vi "XYScan - PLC Controler.vi"() -> ()   [LabVIEW 2018]
uses:
  <vilib>/NI/Modbus Library/API/Wrapper/Create Serial Master.vi
  <vilib>/NI/Modbus Library/API/Master/Modbus Master.lvclass
  <vilib>/NI/Modbus Library/API/Wrapper/API Main.lvlib
panel:
  in  "Distance Mode":bool
  out "Step Y Number":i16=50
  in  "Y Auto Distance":i16=100
  in  "X Auto Distance":i16=200
  in  "Y Distance":u32=200
  in  "X Distance":u32=4
  in  "Y Step":dbl=1.0
  in  "Z Distance":i16=10
  in  "Speed":i32=6
  in  "Home":bool
  in  "Z Up":bool
  in  "Z Down":bool
  in  "Y For":bool
  in  "X Left":bool
  in  "Y Back":bool
  in  "X Right":bool
  in  "VISA":refnum<visa-resource-name>="COM12"
  in  "Stop":bool
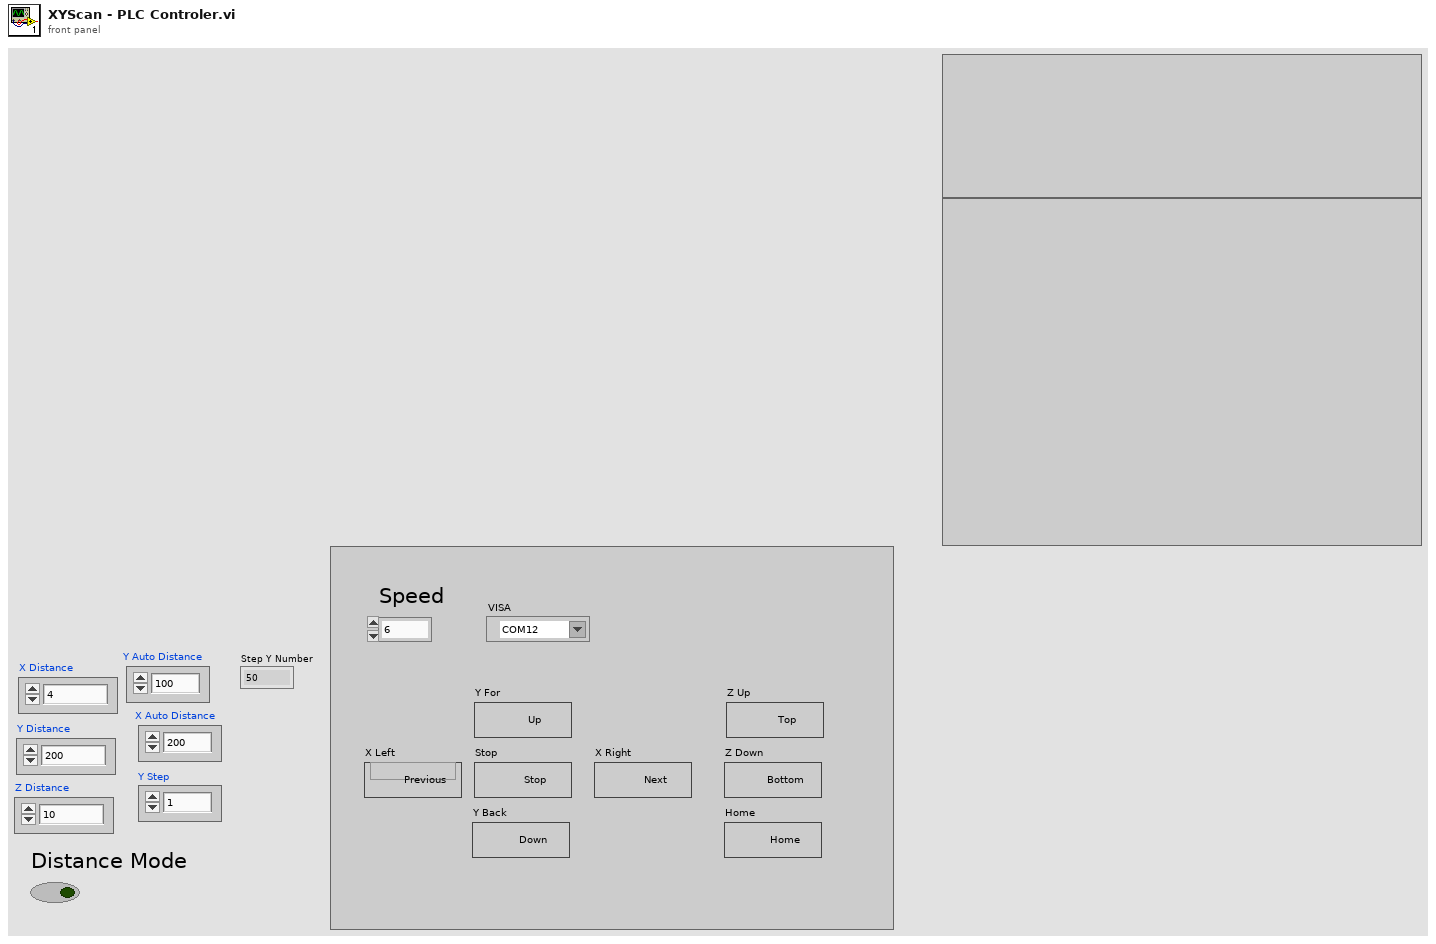
[diagram p1: front panel]
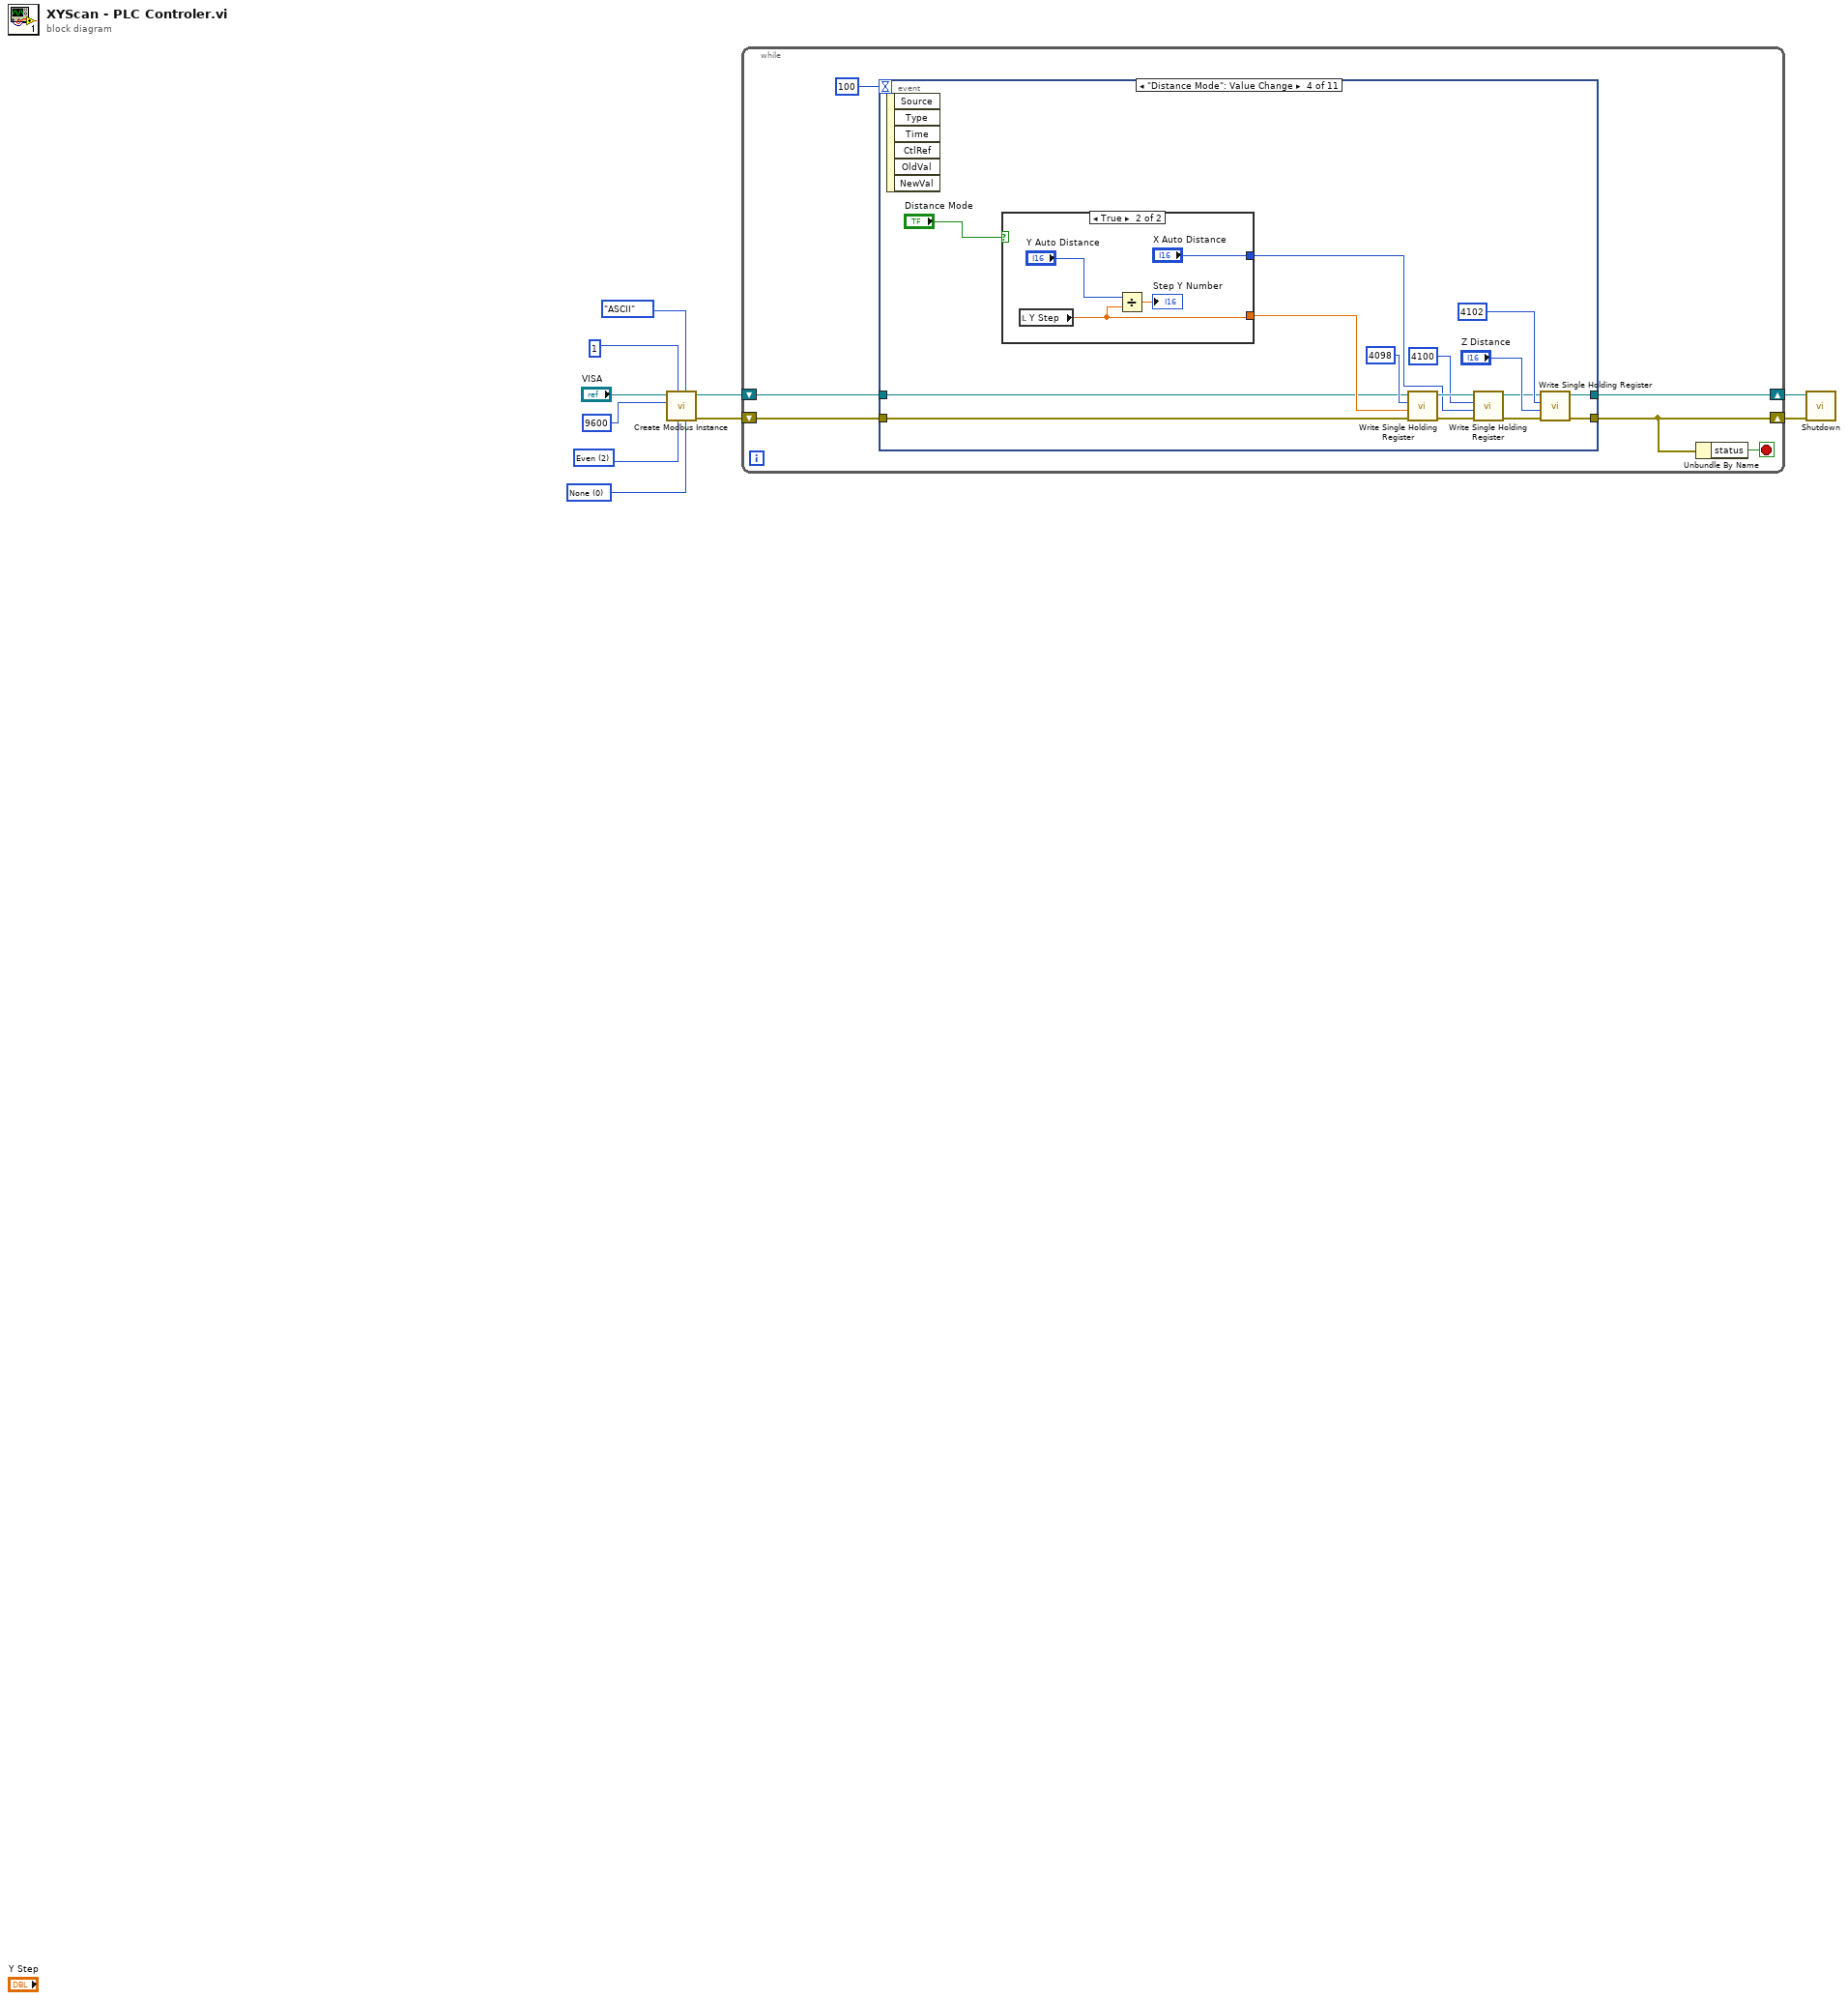
[diagram p0: block diagram]
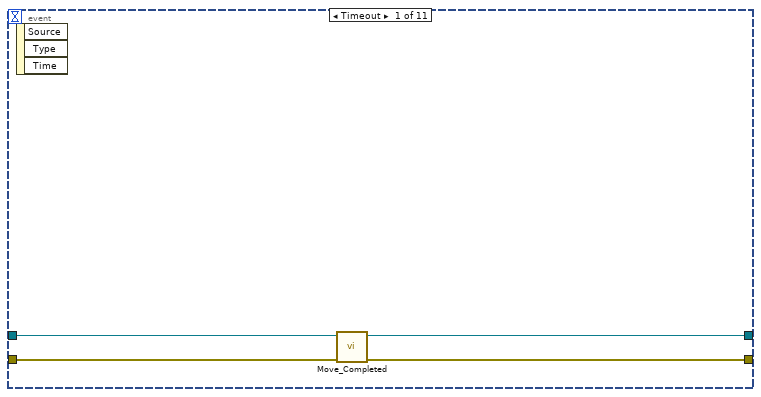
[diagram p2: hidden frame]
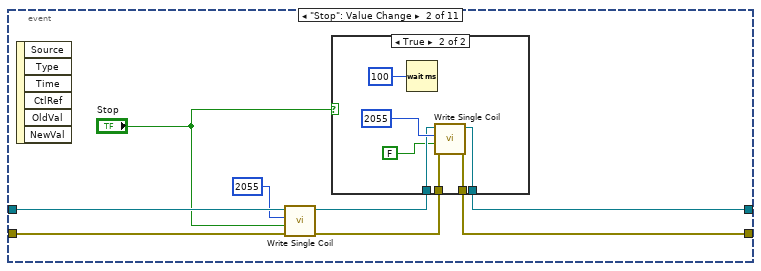
[diagram p3: hidden frame]
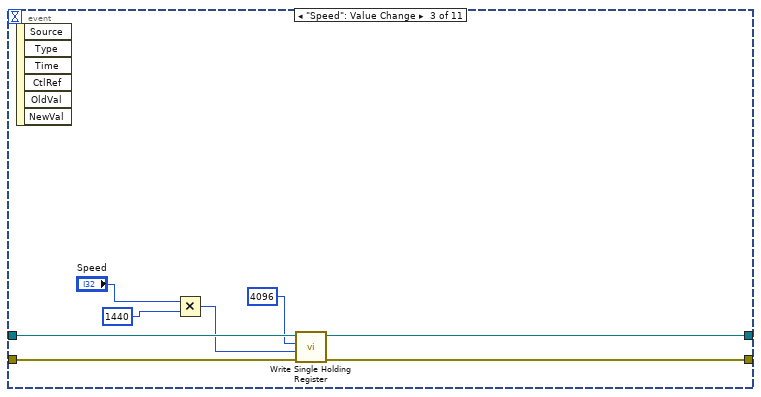
[diagram p5: hidden frame]
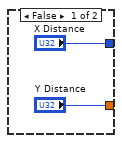
[diagram p6: hidden frame]
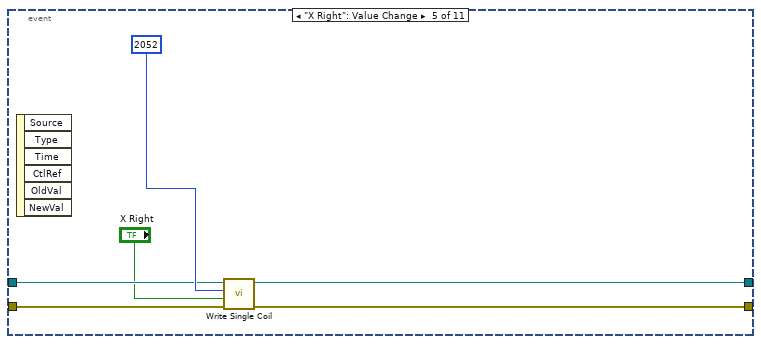
[diagram p7: hidden frame]
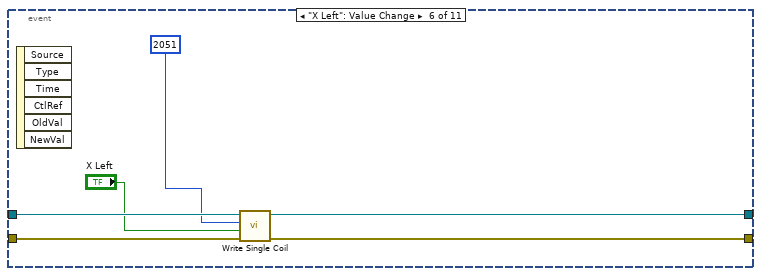
[diagram p8: hidden frame]
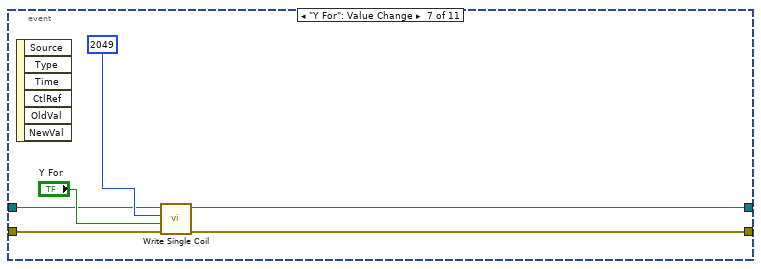
[diagram p9: hidden frame]
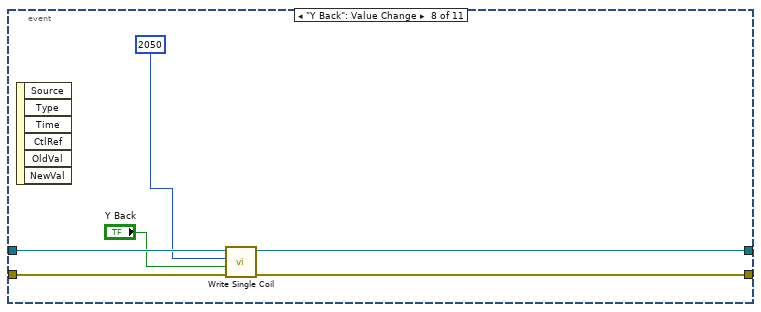
[diagram p10: hidden frame]
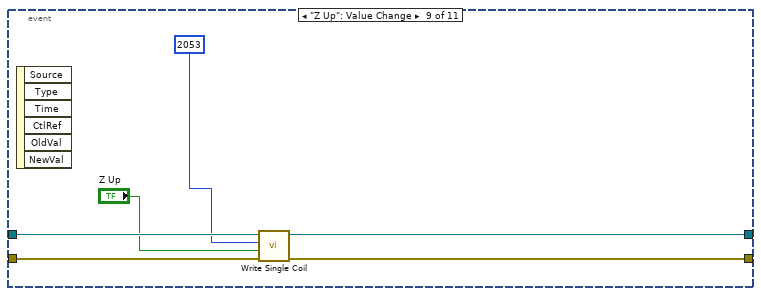
[diagram p11: hidden frame]
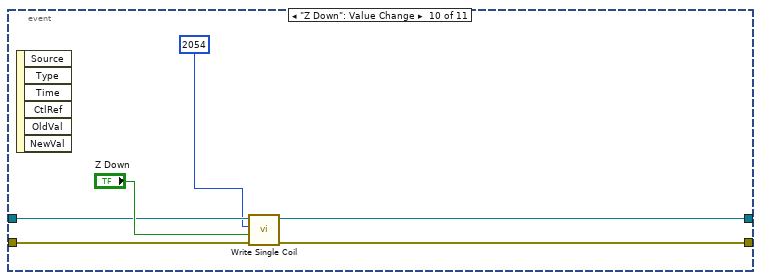
[diagram p12: hidden frame]
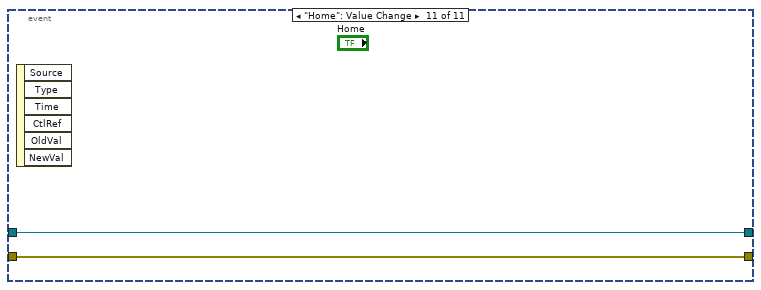
[diagram p13: hidden frame]
diagram:
  w3 = u16 0 items=["None", "XON/XOFF", "RTS/CTS", "XON/XOFF & RTS/CTS", "DTR/DSR", "XON/XOFF & DTR/DSR"] ("flow control (none)")
  w4 = u16 2 items=["None", "Odd", "Even", "Mark", "Space"] ("parity (even)")
  n1 = call-poly <vilib>:"Create Modbus Instance.vi"("flow control (none)"=w3, "serial type"=enum16{"RTU", "ASCII"}."ASCII", "parity (even)"=w4, "unit ID"=u8 1, "baud rate"=u32 9600, "VISA resource name"="VISA") -> ("error out"=w2:errorcluster, "serial master instance"=w1:refnum<class "Modbus Master.lvclass">)  [unwired: 4 in]
  n2 = while {
    shift-right: [w16] -> w10
    shift-left: w1 -> [w12]
    shift-right: [w15] -> w9
    shift-left: w2 -> [w11]
    stop <- w14 stop-if-true
    n3 = event shown="[3] \"Distance Mode\": Value Change" {
      selector: _ -> [_ _ _ _ _ _ _ _ _ _ _]
      dyn-events: _ -> [_ _ _ _ _ _ _ _ _ _ _]
      timeout: 100 -> [_ _ _ _ _ _ _ _ _ _ _]
      tunnel: w12 -> [w18 w28 w45 w47 w71 w78 w82 w90 w96 w98 w104]
      tunnel: [w19 w22 w44 w58 w68 w76 w81 w89 w94 w99 w104] -> w16
      tunnel: w11 -> [w17 w27 w43 w46 w69 w77 w80 w87 w95 w101 w103]
      tunnel: [w20 w21 w42 w57 w67 w75 w79 w88 w93 w100 w103] -> w15
      event Timeout {
        n4 = event-data() -> ()  [unwired: 1 in, 3 out]
        n5 = call "Move_Completed.vi"("error in"=w17, "serial master instance"=w18) -> ("error out"=w20:errorcluster, "Modbus master out"=w19:refnum<class "Modbus Master.lvclass">)  [unwired: 5 in]
      }
      event "Stop": Value Change {
        n6 = event-data() -> ()  [unwired: 1 in, 6 out]
        n7 = call-dynamic "Write Single Coil.vi"("error in"=w27, "coil to write"="Stop", "address"=u16 2055, "Modbus master in"=w28) -> ("error out"=w24:errorcluster, "Modbus master out"=w23:refnum<class "Modbus Master.lvclass">)  [unwired: 6 in]
        n8 = case shown="True" "Stop" {
          tunnel: w23 -> [w29 w35]
          tunnel: w24 -> [w30 w34]
          tunnel: [w29 w33] -> w22
          tunnel: [w30 w32] -> w21
          frame False {
          }
          frame True {
            n9 = Wait (ms)(milliseconds to wait=u32 100 ("millisecond timer value")) -> ()  [unwired: 1 out]
            n10 = call-dynamic "Write Single Coil.vi"("error in"=w34, "coil to write"=FALSE, "address"=u16 2055, "Modbus master in"=w35) -> ("error out"=w32:errorcluster, "Modbus master out"=w33:refnum<class "Modbus Master.lvclass">)  [unwired: 6 in]
          }
        }
      }
      event "Speed": Value Change {
        n11 = event-data() -> ()  [unwired: 1 in, 6 out]
        n12 = Multiply(x="Speed", y=i16 1440 ("Speed (mm/s)")) -> (x*y=w39:i32)
        n13 = call-dynamic "Write Single Holding Register.vi"("error in"=w43, "register to write"=w39, "address"=u16 4096, "Modbus master in"=w45) -> ("error out"=w42:errorcluster, "Modbus master out"=w44:refnum<class "Modbus Master.lvclass">)  [unwired: 6 in]
      }
      event "Distance Mode": Value Change {
        n14 = event-data() -> ()  [unwired: 1 in, 6 out]
        n15 = case shown="True" "Distance Mode" {
          tunnel: ["Y Distance" w63] -> w53
          tunnel: ["X Distance" "X Auto Distance"] -> w54
          frame False {
          }
          frame True {
            n16 = local read "Y Step"() -> (w63:dbl)
            n17 = Divide(x="Y Auto Distance", y=w63) -> (x/y=→"Step Y Number":dbl)
          }
        }
        n18 = call-dynamic "Write Single Holding Register.vi"("error in"=w46, "register to write"=w53, "address"=u16 4098, "Modbus master in"=w47) -> ("error out"=w55:errorcluster, "Modbus master out"=w56:refnum<class "Modbus Master.lvclass">)  [unwired: 6 in]
        n19 = call-dynamic "Write Single Holding Register.vi"("error in"=w55, "register to write"=w54, "address"=u16 4100, "Modbus master in"=w56) -> ("error out"=w48:errorcluster, "Modbus master out"=w49:refnum<class "Modbus Master.lvclass">)  [unwired: 6 in]
        n20 = call-dynamic "Write Single Holding Register.vi"("error in"=w48, "register to write"="Z Distance", "address"=u16 4102, "Modbus master in"=w49) -> ("error out"=w57:errorcluster, "Modbus master out"=w58:refnum<class "Modbus Master.lvclass">)  [unwired: 6 in]
      }
      event "X Right": Value Change {
        n21 = event-data() -> ()  [unwired: 1 in, 6 out]
        n22 = call-dynamic "Write Single Coil.vi"("error in"=w69, "coil to write"="X Right", "address"=u16 2052, "Modbus master in"=w71) -> ("error out"=w67:errorcluster, "Modbus master out"=w68:refnum<class "Modbus Master.lvclass">)  [unwired: 6 in]
      }
      event "X Left": Value Change {
        n23 = event-data() -> ()  [unwired: 1 in, 6 out]
        n24 = call-dynamic "Write Single Coil.vi"("error in"=w77, "coil to write"="X Left", "address"=u16 2051, "Modbus master in"=w78) -> ("error out"=w75:errorcluster, "Modbus master out"=w76:refnum<class "Modbus Master.lvclass">)  [unwired: 6 in]
      }
      event "Y For": Value Change {
        n25 = event-data() -> ()  [unwired: 1 in, 6 out]
        n26 = call-dynamic "Write Single Coil.vi"("error in"=w80, "coil to write"="Y For", "address"=u16 2049, "Modbus master in"=w82) -> ("error out"=w79:errorcluster, "Modbus master out"=w81:refnum<class "Modbus Master.lvclass">)  [unwired: 6 in]
      }
      event "Y Back": Value Change {
        n27 = event-data() -> ()  [unwired: 1 in, 6 out]
        n28 = call-dynamic "Write Single Coil.vi"("error in"=w87, "coil to write"="Y Back", "address"=u16 2050, "Modbus master in"=w90) -> ("error out"=w88:errorcluster, "Modbus master out"=w89:refnum<class "Modbus Master.lvclass">)  [unwired: 6 in]
      }
      event "Z Up": Value Change {
        n29 = event-data() -> ()  [unwired: 1 in, 6 out]
        n30 = call-dynamic "Write Single Coil.vi"("error in"=w95, "coil to write"="Z Up", "address"=u16 2053, "Modbus master in"=w96) -> ("error out"=w93:errorcluster, "Modbus master out"=w94:refnum<class "Modbus Master.lvclass">)  [unwired: 6 in]
      }
      event "Z Down": Value Change {
        n31 = event-data() -> ()  [unwired: 1 in, 6 out]
        n32 = call-dynamic "Write Single Coil.vi"("error in"=w101, "coil to write"="Z Down", "address"=u16 2054, "Modbus master in"=w98) -> ("error out"=w100:errorcluster, "Modbus master out"=w99:refnum<class "Modbus Master.lvclass">)  [unwired: 6 in]
      }
      event "Home": Value Change {
        n33 = event-data() -> ()  [unwired: 1 in, 6 out]
      }
    }
    n34 = Unbundle By Name(w15) -> ("status"=w14:bool)
  }
  n35 = call-dynamic "Shutdown.vi"("error in"=w9, "Modbus master in"=w10) -> ()  [unwired: 9 in, 1 out]
